vi "ReadFromTextFile_v3.vi"(6 "Display Data":bool=TRUE, 7 "Convert Phase to Radians":bool, 8 "Convert Amplitude to dB":bool, 9 "Skip First N Lines":i32=48, 10 "name or relative path":path=path "C:/Users/LAV-UFSC/OneDrive - UFSC/Documents/LAV - TCC/Dados-Experimentos/5-6-23/guidaoCentroAte500.txt") -> (0 "Phase":dbl[][](array[numeric]), 1 "Magnitude":dbl[][](array[numeric]), 2 "Phase":cluster{dbl[], dbl[]}, 3 "Magnitude":cluster{dbl[], dbl[]})   [LabVIEW 2022 SP3]
uses:
  <vilib>/Utility/file.llb/Read Delimited Spreadsheet (DBL).vi
panel:
  in  "Max. Freq.":i32=500
  in  "Output Type":bool
  out "Phase":cluster{"Array":dbl[], "Array":dbl[]}(graph) caption="Amplitude [Hz]"
  out "Magnitude":cluster{"Array":dbl[], "Array":dbl[]}(graph) caption="Amplitude [Hz]"
  out "number of rows":i32
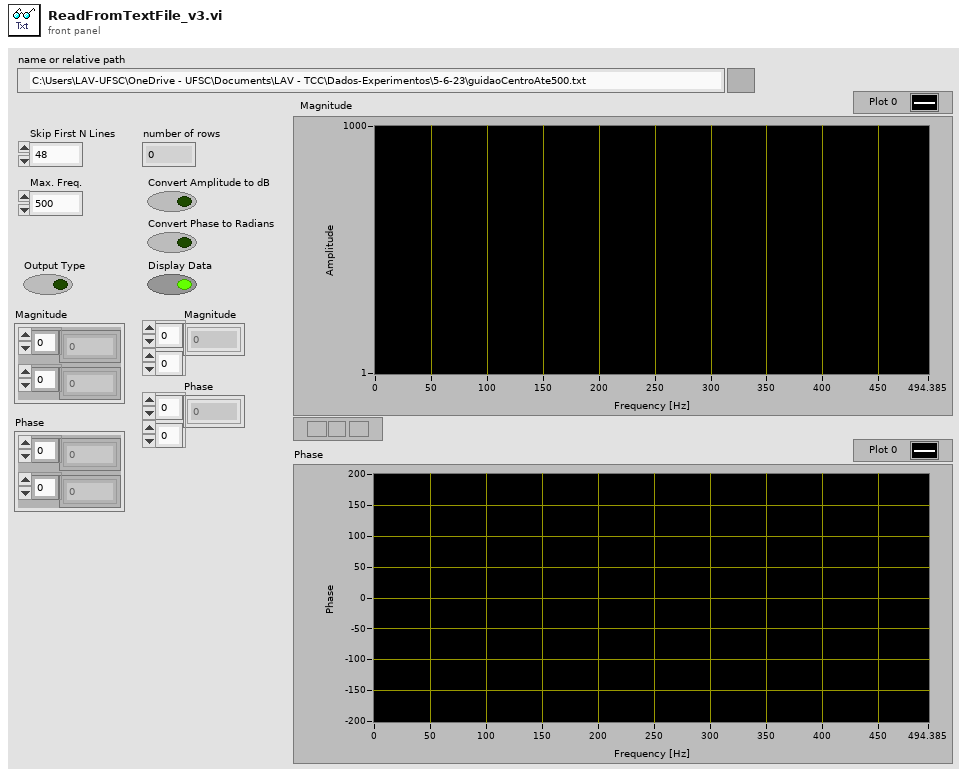
[diagram p1: front panel]
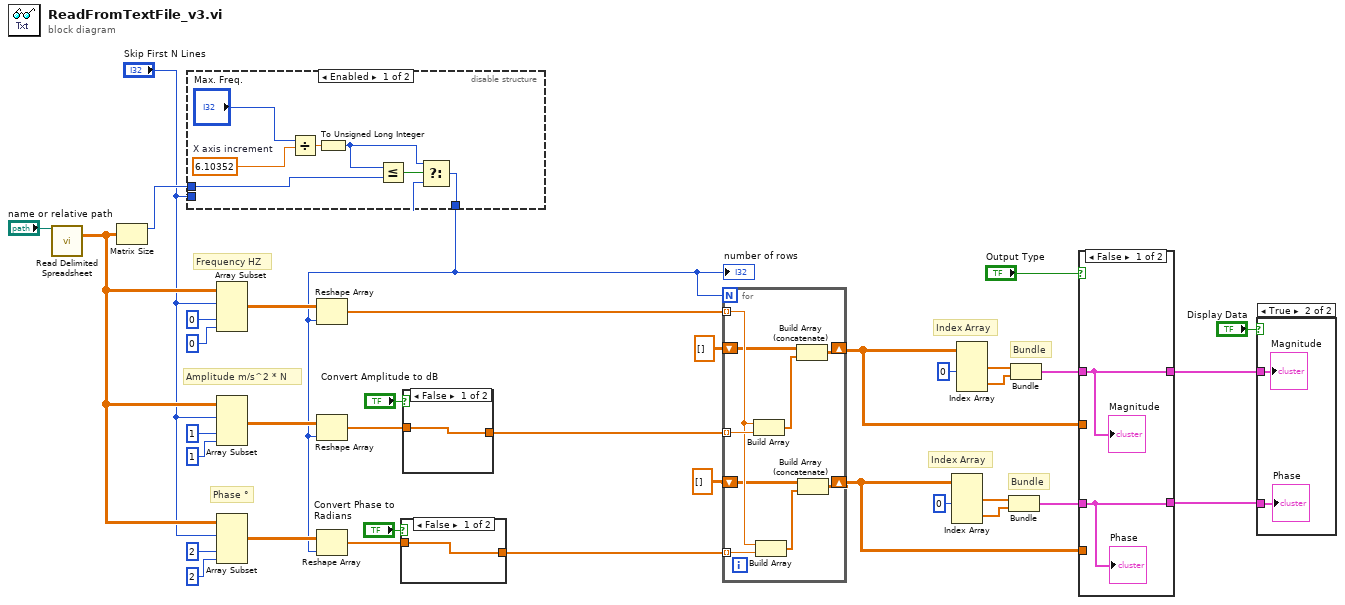
[diagram p0: block diagram]
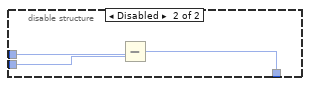
[diagram p2: hidden frame]
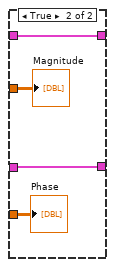
[diagram p3: hidden frame]
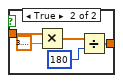
[diagram p5: hidden frame]
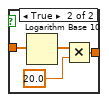
[diagram p6: hidden frame]
diagram:
  # "Index Array"
  # "Bundle"
  # "Index Array"
  # "Bundle"
  # "Phase °"
  # "Amplitude m/s^2 * N"
  # "Frequency HZ"
  n1 = call-poly <vilib>:"Read Delimited Spreadsheet.vi"("file path (dialog if empty)"="name or relative path") -> ("all rows"=w28:dbl[][])  [unwired: 9 in, 5 out]
  n2 = Matrix Size(0:w28) -> (1:w3:i32)  [unwired: 1 out]
  n3 = disable-structure shown="Enabled" {
    disable-tunnel: w3 -> [w43 w47]
    disable-tunnel: [w42 w45] -> w2
    disable-tunnel: "Skip First N Lines" -> [_ w46]
    frame Enabled {
      w41 = 6.10352  # X axis increment
      n4 = Divide(x="Max. Freq.", y=w41) -> (x/y=w39:dbl)
      n5 = To Unsigned Long Integer(number=w39) -> (unsigned 32bit integer=w38:u32)
      n6 = Less Or Equal?(x=w38, y=w43) -> (x <= y?=w44:bool)
      n7 = Select(t=w38, s=w44, f=w43) -> (s? t:f=w42:u32)
    }
    frame Disabled {
      n8 = Subtract(x=w47, y=w46) -> (x-y=w45:i32)
    }
  }
  "number of rows" <- w2
  n9 = Array Subset(array=w28, index (row)="Skip First N Lines", index (col)=0 ("column 1"), length (col)=0 ("column N")) -> (w30:dbl[][])  [unwired: 1 in]
  n10 = Array Subset(array=w28, index (row)="Skip First N Lines", index (col)=1 ("column 1"), length (col)=1 ("column N")) -> (w29:dbl[][])  [unwired: 1 in]
  n11 = Array Subset(array=w28, index (row)="Skip First N Lines", index (col)=2 ("column 1"), length (col)=2 ("column N")) -> (w17:dbl[][])  [unwired: 1 in]
  n12 = Reshape Array(w30, w2) -> (w16:dbl[])
  n13 = Reshape Array(w29, w2) -> (w15:dbl[])
  n14 = Reshape Array(w17, w2) -> (w13:dbl[])
  n15 = case shown="False" "Convert Phase to Radians" {
    tunnel: w13 -> [w48 w52]
    tunnel: [w48 w49] -> w12
    frame False {
    }
    frame True {
      n16 = Multiply(x=w52, y=3.141592653589793) -> (x*y=w53:dbl[])
      n17 = Divide(x=w53, y=180) -> (x/y=w49:dbl[])
    }
  }
  n18 = case shown="False" "Convert Amplitude to dB" {
    tunnel: [w54 w56] -> w23
    tunnel: w15 -> [w54 w55]
    frame False {
    }
    frame True {
      n19 = Logarithm Base 10(1:w55) -> (0:w57:dbl[])
      n20 = Multiply(x=w57, y=20.0) -> (x*y=w56:dbl[])
    }
  }
  n21 = for {
    N: w2 -> [_]
    tunnel: w16 -> [w65] mode=indexing
    tunnel: w23 -> [w66] mode=indexing
    tunnel: w12 -> [w67] mode=indexing
    shift-right: [w62] -> w9
    shift-left: dbl[][] [] -> [w64]
    shift-right: [w61] -> w18
    shift-left: dbl[][] [] -> [w60]
    n22 = Build Array(w65, w66) -> (w63:dbl[])
    n23 = Build Array(w65, w67) -> (w59:dbl[])
    n24 = Build Array (concatenate)(w64, w63) -> (w62:dbl[][])
    n25 = Build Array (concatenate)(w60, w59) -> (w61:dbl[][])
  }
  n26 = Index Array(array=w18, index (col) #1=0 ("disabled index (col)")) -> (element #1=w19:dbl[], element #2=w20:dbl[])  [unwired: 3 in]
  n27 = Index Array(array=w9, index (col) #1=0 ("disabled index (col)")) -> (element #1=w24:dbl[], element #2=w25:dbl[])  [unwired: 3 in]
  n28 = Bundle(w19, w20) -> (w7:cluster{dbl[], dbl[]})  [unwired: 1 in]
  n29 = Bundle(w24, w25) -> (w5:cluster{dbl[], dbl[]})  [unwired: 1 in]
  n30 = case shown="False" "Output Type" {
    tunnel: w18 -> [_ w73]
    tunnel: w9 -> [_ w72]
    tunnel: w7 -> [w68 w71]
    tunnel: [w68 w71] -> w6
    tunnel: w5 -> [w69 w70]
    tunnel: [w69 w70] -> w4
    frame False {
      "Magnitude" <- w69
      "Phase" <- w68
    }
    frame True {
      "Phase" <- w73
      "Magnitude" <- w72
    }
  }
  n31 = case shown="True" "Display Data" {
    tunnel: w4 -> [_ w75]
    tunnel: w6 -> [_ w74]
    frame False {
    }
    frame True {
      "Magnitude" <- w75
      "Phase" <- w74
    }
  }
